vi "SetOutputEnable.vi"(8 "ErrorArray In":errorcluster[](array[cluster]), 10 "clFrontPanelControlRefs":T1, 11 "NISTBus In":refnum<class "NISTBus.lvclass">) -> (0 "ErrorArray Out":errorcluster[](array[cluster]), 3 "NISTBus Out":refnum<class "NISTBus.lvclass">)   [LabVIEW 2014, in "Bus.lvlib" / "NISTBus.lvclass"]
uses:
  NISTBus.lvclass
  Framework/FrontPanel/TypeDefs/clFrontPanelControlRefs.ctl
  FGenPlugins/MyPluginBaseClass/TypeDef/PluginParams.ctl
  WfrmGenerator/WfrmPlugins/EventPluginBaseClass/TypeDefs/dblEvtSignalArray.ctl
  FGenPlugins/MyPluginBaseClass/TypeDef/CreateArbWfrmParams.ctl
  WfrmGenerator/WfrmPlugins/EventPluginBaseClass/TypeDefs/clEvtConfig.ctl
  WfrmGenerator/WfrmModule/PublicAPI/Arguments/Requests/dblEvtParams.ctl
  FGenPlugins/MyPluginBaseClass/TypeDef/ConfigArbWfrmParams.ctl
  FGenPlugins/MyPluginBaseClass/TypeDef/TriggerParams.ctl
  <userlib>/NIST/NISTErrorLib/NISTErrorLib.lvlib
  FGenPlugins/MyPluginBaseClass/NISTFGenPluginsBase.lvclass
  WfrmGenerator/WfrmPlugins/EventPluginBaseClass/BaseWfrmPlugin.lvclass
  Framework/TestFramework.lvlib
  WfrmGenerator/WfrmModule/WfrmModule.lvlib
panel:
  # "When you add a control \non the front panel, add a\nreference for it in this\ntype def.  This cluster\nwill hold all of the refer-\nences to the front panel\ncontrols in order to pass\nthese control references \nto subvis."
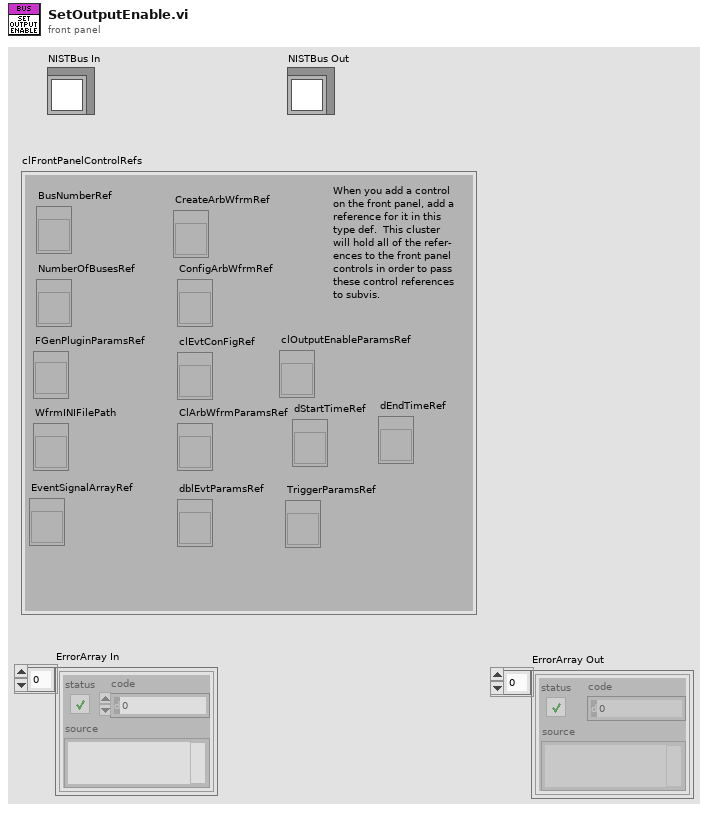
[diagram p1: front panel]
types:
  T1 = typedef "TestFramework.lvlib/clFrontPanelControlRefs.ctl" = cluster{"BusNumberRef":refnum<vi>, "NumberOfBusesRef":refnum<vi>, "FGenPluginParamsRef":refnum<vi>, "WfrmINIFilePath":refnum<vi>, "EventSignalArrayRef":refnum<vi>, "CreateArbWfrmRef":refnum<vi>, "clEvtConFigRef":refnum<vi>, "dblEvtParamsRef":refnum<vi>, "clOutputEnableParamsRef":refnum<vi>, "ConfigArbWfrmRef":refnum<vi>, "ClArbWfrmParamsRef":refnum<vi>, "dStartTimeRef":refnum<vi>, "dEndTimeRef":refnum<vi>, "TriggerParamsRef":refnum<vi>}
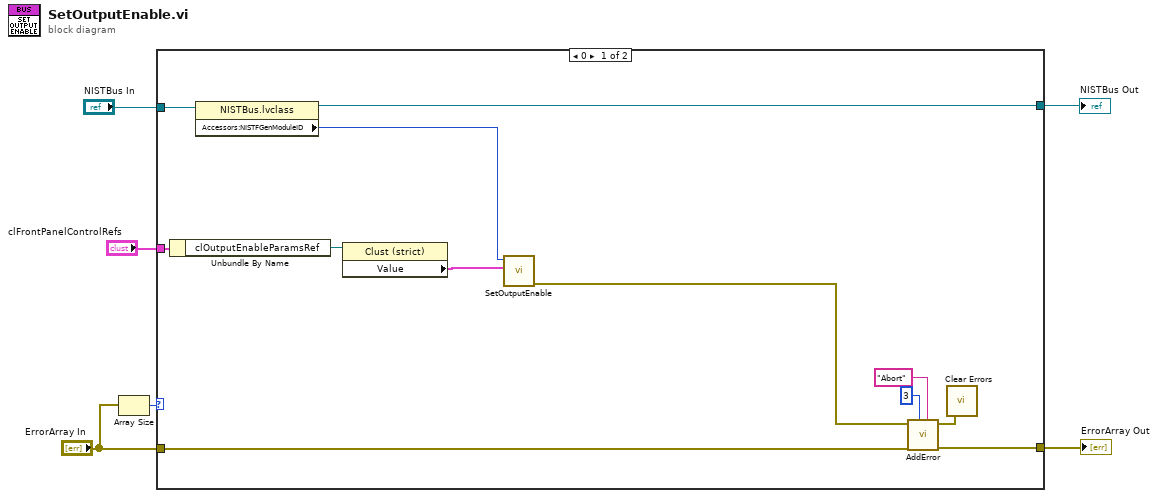
[diagram p0: block diagram]
diagram:
  n1 = Array Size(array="ErrorArray In") -> (size(s)=w6:i32)
  n2 = case shown="0" w6 {
    tunnel: "ErrorArray In" -> [w15 w20]
    tunnel: [w14 w20] -> w4
    tunnel: "NISTBus In" -> [w13 w19]
    tunnel: "clFrontPanelControlRefs" -> [w11 _]
    tunnel: [w12 w19] -> w1
    frame 0 {
      n3 = Unbundle By Name(w11) -> ("clOutputEnableParamsRef"=w10:refnum<vi>)
      n4 = property class="NISTBus.lvclass"(reference=w13) -> (reference out=w12:refnum<class "NISTBus.lvclass">, "Accessors:NISTFGenModuleID"=w7:i32)  [unwired: 1 in, 1 out]
      n5 = property class="Clust (strict)"(reference=w10) -> ("Value"=w9:cluster{"sName":string, "bEnabled":bool})  [unwired: 1 in, 2 out]
      n6 = call "SetOutputEnable.vi"("OutputEnableParams"=w9, "ModuleID"=w7) -> ("error out"=w8:errorcluster)  [unwired: 9 in]
      n7 = call <userlib>:"AddError.vi"("Severity"="Abort" ("String"), "Priority"=u8 3, "ErrorArray"=w15, "error in (no error)"=w8) -> ("ErrorArray"=w14:errorcluster[], "error out"=w16:errorcluster)  [unwired: 6 in]
      n8 = call <vilib>:"Clear Errors.vi"("error in (no error)"=w16) -> ()  [unwired: 5 in, 2 out]
    }
    frame 1, Default {
    }
  }
  "NISTBus Out" <- w1
  "ErrorArray Out" <- w4
